vi "Update Errors.vi"(8 "error in (no error)":errorcluster, 10 "error_info":T1[](array[typedef]), 11 "Error MCLB reference in":refnum<vi>) -> (0 "error out":errorcluster, 3 "Error MCLB reference out":refnum<vi>)   [LabVIEW 2021, in "CIF_UI.lvclass"]
uses:
  CIF_UI.lvclass
  CIFPluginManager/CIFPluginManager/gRPC/CIF_Manager_client/RPC Messages/cif_manager_ErrorInfo.ctl
  CIF_UI.lvclass/CIF_UI.ctl
  CIFPluginManager/CIFPluginManager/gRPC/CIF_Manager_client/CIF_Manager_client.lvlib
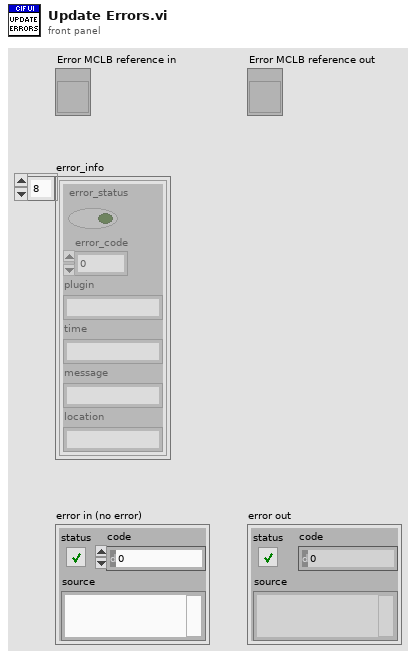
[diagram p1: front panel]
types:
  T1 = typedef "CIF_Manager_client.lvlib/cif_manager_ErrorInfo.ctl" = cluster{"error_status":bool, "error_code":i32, "plugin":string, "time":string, "message":string, "location":string}
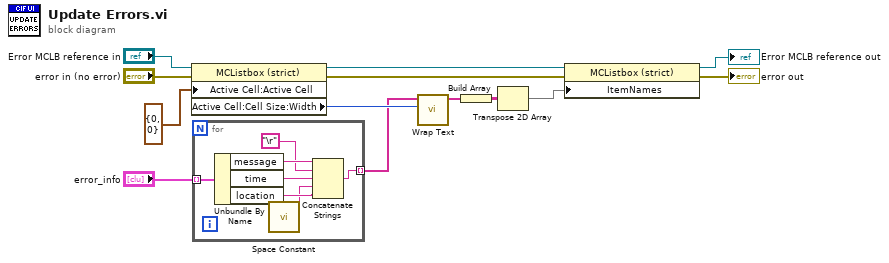
[diagram p0: block diagram]
diagram:
  n1 = property on="Property Node" class="MCListbox (strict)"(reference="Error MCLB reference in", error in="error in (no error)", "Active Cell:Active Cell"=cluster{"Row":i32, "Column":i32} {"Row"=0, "Column"=0} ("Active Cell")) -> (reference out=w2:refnum<vi>, error out=w4:errorcluster, "Active Cell:Cell Size:Width"=w11:u32)
  n2 = for {
    tunnel: "error_info" -> [w20] mode=indexing
    tunnel: [w18] -> w10 mode=indexing
    n3 = Unbundle By Name(w20) -> ("message"=w19:string, "time"=w16:string, "location"=w17:string)
    n4 = call <vilib>:"Space Constant.vi"() -> ("String"=w14:string)
    n5 = Concatenate Strings(w19, "\r", w16, w14, w17) -> (w18:string)
  }
  n6 = call "Wrap Text.vi"("width"=w11, "item names"=w10) -> ("item names with wrapping"=w9:string[])  [unwired: 8 in, 1 out]
  n7 = Build Array(w9) -> (w8:string[][])
  n8 = Transpose 2D Array(2D array=w8) -> (transposed array=w7:string[][])
  n9 = property class="MCListbox (strict)"(reference=w2, error in=w4, "ItemNames"=w7) -> (reference out=→"Error MCLB reference out":refnum<vi>, error out=→"error out":errorcluster)
